vi "ShutDown5Panes.vi"(8 "error in (no error)":errorcluster, 11 "PentaPanesGUI in":refnum<class "PentaPanes.lvclass">) -> (0 "error out":errorcluster)   [LabVIEW 2022 SP3, in "PentaPanesLibrary.lvlib" / "PentaPanes.lvclass"]
doc: "ShutDownPentaPanes\nThis VI clears and closes PentaPanes object."
uses:
  PentaPanes.lvclass
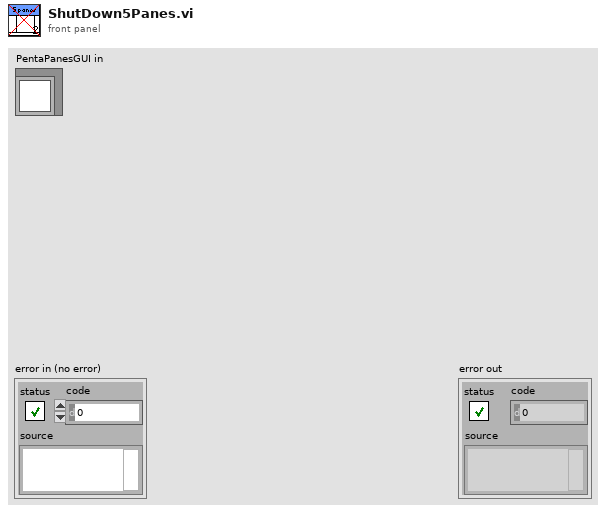
[diagram p1: front panel]
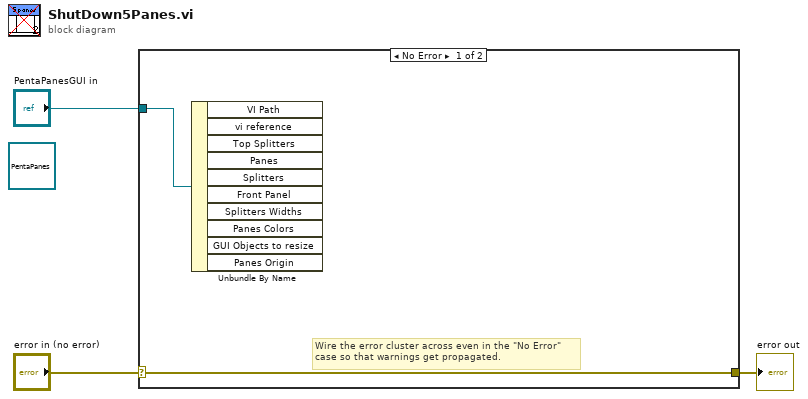
[diagram p0: block diagram]
diagram:
  (unwired) refnum<class "PentaPanes.lvclass"> refnum ("PentaPanesGUI.lvclass")
  n1 = case shown="No Error" "error in (no error)" {
    selector: "error in (no error)" -> [w5 w6]
    tunnel: [w5 w6] -> w2
    tunnel: "PentaPanesGUI in" -> [w4 _]
    frame No Error {
      # "Wire the error cluster across even in the \"No Error\"\ncase so that warnings get propagated."
      n2 = Unbundle By Name(w4) -> ()  [unwired: 10 out]
    }
    frame Error {
    }
  }
  "error out" <- w2
